vi "create_image1.vi"(8 "error in":errorcluster, 11 "base path":path) -> (0 "error out":errorcluster, 3 "path":path)   [LabVIEW 2018]
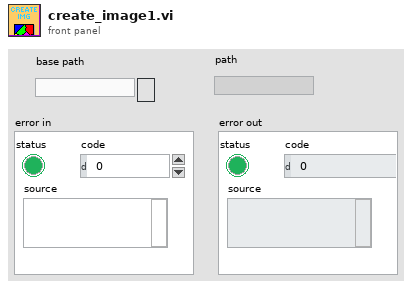
[diagram p1: front panel]
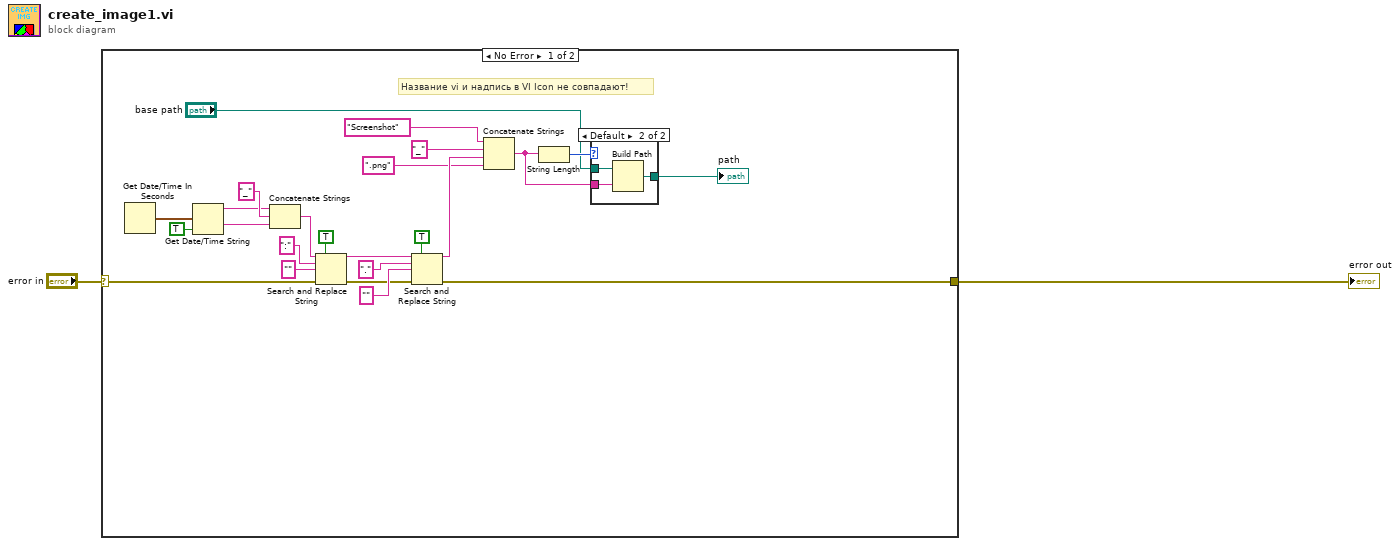
[diagram p0: block diagram]
diagram:
  n1 = case shown="No Error" "error in" {
    selector: "error in" -> [w7 w31]
    tunnel: [w4 w31] -> w2
    frame No Error {
      # "Название vi и надпись в VI Icon не совпадают!"
      n2 = Get Date/Time In Seconds() -> (seconds since 1Jan1904=w13:timestamp)
      n3 = Get Date/Time String(seconds (now)=w13, want seconds? (F)=TRUE) -> (date string=w14:string, time string=w22:string)  [unwired: 1 in]
      n4 = Concatenate Strings(w14, "_" ("string"), w22) -> (w15:string)
      n5 = Search and Replace String(replace all?=TRUE, input string=w15, search string=":", replace string="" ("replace string (\"\")"), error in=w7) -> (result string=w18:string, error out=w8:errorcluster)  [unwired: 3 in, 2 out]
      n6 = Search and Replace String(replace all?=TRUE, input string=w18, search string=".", replace string="" ("replace string (\"\")"), error in=w8) -> (result string=w10:string, error out=w4:errorcluster)  [unwired: 3 in, 2 out]
      n7 = Concatenate Strings("Screenshot" ("name or relative path"), "_" ("name or relative path"), w10, ".png" ("string")) -> (w26:string)
      n8 = String Length(string=w26) -> (length=w25:i32)
      n9 = case shown="Default" w25 {
        tunnel: [w27 w30] -> w9
        tunnel: "base path" -> [w27 w29]
        tunnel: w26 -> [_ w28]
        frame 0 {
        }
        frame Default {
          n10 = Build Path(base path=w29, name or relative path=w28) -> (appended path=w30:path)
        }
      }
      "path" <- w9
    }
    frame Error {
    }
  }
  "error out" <- w2
